vi "ManipLED_Overide.vi"(3 "Instruction String":string) -> (0 "Error Out":errorcluster, 1 "Advance Trigger":bool)   [LabVIEW 2019]
uses:
  SafeParser_String.vi
  outputs.vi
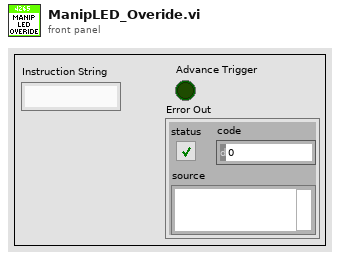
[diagram p1: front panel]
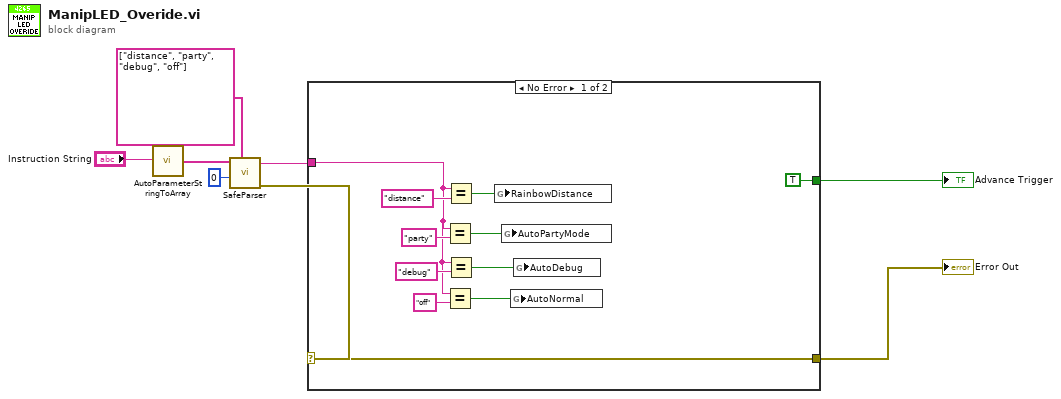
[diagram p0: block diagram]
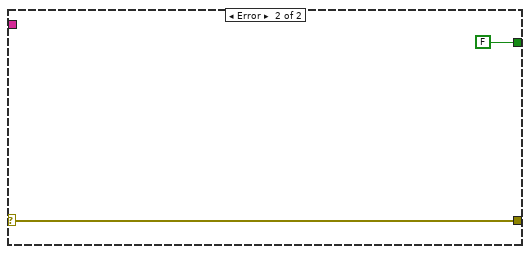
[diagram p2: hidden frame]
diagram:
  n1 = call "AutoParameterStringToArray.vi"("Parameter String"="Instruction String") -> ("Parsed Parameters"=w5:string[])
  n2 = call-poly "SafeParser.vi"("Allowed Values"=string[] ["distance", "party", "debug", "off"], "Array Index"=0 ("Parameter Index"), "String Array"=w5) -> ("Error Out"=w3:errorcluster, "Typecast Value"=w4:string)  [unwired: 7 in]
  n3 = case shown="No Error" w3 {
    selector: w3 -> [w18 w20]
    tunnel: [TRUE ("Advance Trigger") FALSE ("Advance Trigger")] -> w8
    tunnel: [w18 w20] -> w7
    tunnel: w4 -> [w9 _]
    frame No Error {
      n4 = Equal?(x=w9, y="party") -> (x = y?=w14:bool)
      n5 = Equal?(x=w9, y="off") -> (x = y?=w10:bool)
      n6 = Equal?(x=w9, y="distance") -> (x = y?=w16:bool)
      n7 = Equal?(x=w9, y="debug") -> (x = y?=w12:bool)
      n8 = global write "outputs.vi" "RainbowDistance"(w16) -> ()
      n9 = global write "outputs.vi" "AutoPartyMode"(w14) -> ()
      n10 = global write "outputs.vi" "AutoNormal"(w10) -> ()
      n11 = global write "outputs.vi" "AutoDebug"(w12) -> ()
    }
    frame Error {
    }
  }
  "Advance Trigger" <- w8
  "Error Out" <- w7
